vi "uPolicy_TopicIsRelevant.vi"(8 "error in (no error)":errorcluster, 10 "Observed Topic (Lower Case)":string, 11 "wildcards in":refnum<class "wildcards.lvclass">) -> (0 "error out":errorcluster, 2 "Relevant?":bool, 3 "wildcards out":refnum<class "wildcards.lvclass">)   [LabVIEW 2023, in "uFramework_pack_uPolicy.lvlib" / "wildcards.lvclass"]
uses:
  wildcards.lvclass
  wildcards.lvclass/wildcards.ctl
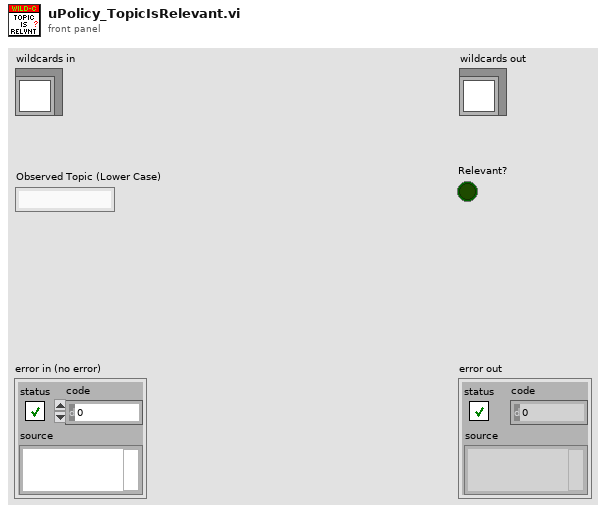
[diagram p1: front panel]
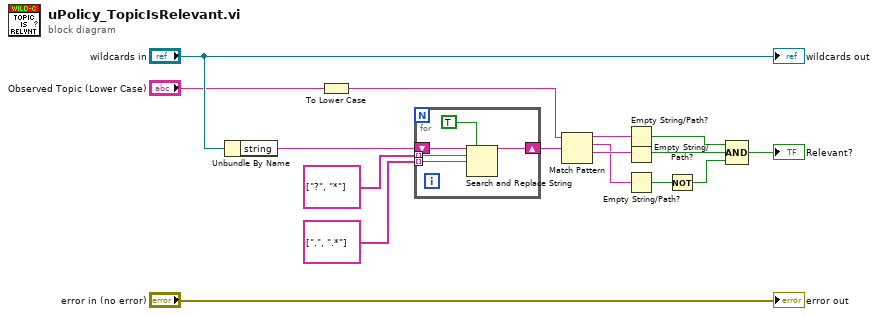
[diagram p0: block diagram]
diagram:
  n1 = Unbundle By Name("wildcards in") -> ("string"=w4:string)
  n2 = To Lower Case(string="Observed Topic (Lower Case)") -> (all lower case string=w1:string)
  n3 = for {
    shift-right: [w20] -> w7
    shift-left: w4 -> [w21]
    tunnel: string[] ["?", "*"] -> [w18] mode=indexing
    tunnel: string[] [".", ".*"] -> [w17] mode=indexing
    n4 = Search and Replace String(replace all?=TRUE ("replace all? (F)"), input string=w21, search string=w18, replace string=w17) -> (result string=w20:string)  [unwired: 4 in, 3 out]
  }
  n5 = Match Pattern(string=w1, regular expression=w7) -> (before substring=w14:string, match substring=w12:string, after substring=w13:string)  [unwired: 1 in, 1 out]
  n6 = Empty String/Path?(string/path=w14) -> (empty?=w11:bool)
  n7 = Empty String/Path?(string/path=w13) -> (empty?=w10:bool)
  n8 = Empty String/Path?(string/path=w12) -> (empty?=w9:bool)
  n9 = Not(x=w9) -> (.not. x?=w8:bool)
  n10 = Compound Arithmetic op=AND(w11, w10, w8) -> (→"Relevant?":bool)
  "error out" <- "error in (no error)"
  "wildcards out" <- "wildcards in"
